vi "Periodic Tasks.vi"(8 "error in":errorcluster) -> ()   [LabVIEW 2020]
doc: "This VI runs in parallel to other tasks. It can contain as many user-defined periodic loops as you need. These can carry out PID or other sorts of timed response."
uses:
  <vilib>/Rock Robotics/WPI/Utilities/WPI_GetSetVariantRefNum.vi
panel:
  out "Temperature Chart":u8(graph)
  out "Output Chart":dbl(graph)
  out "Current Chart":dbl(graph)
  out "Voltage Chart":dbl(graph)
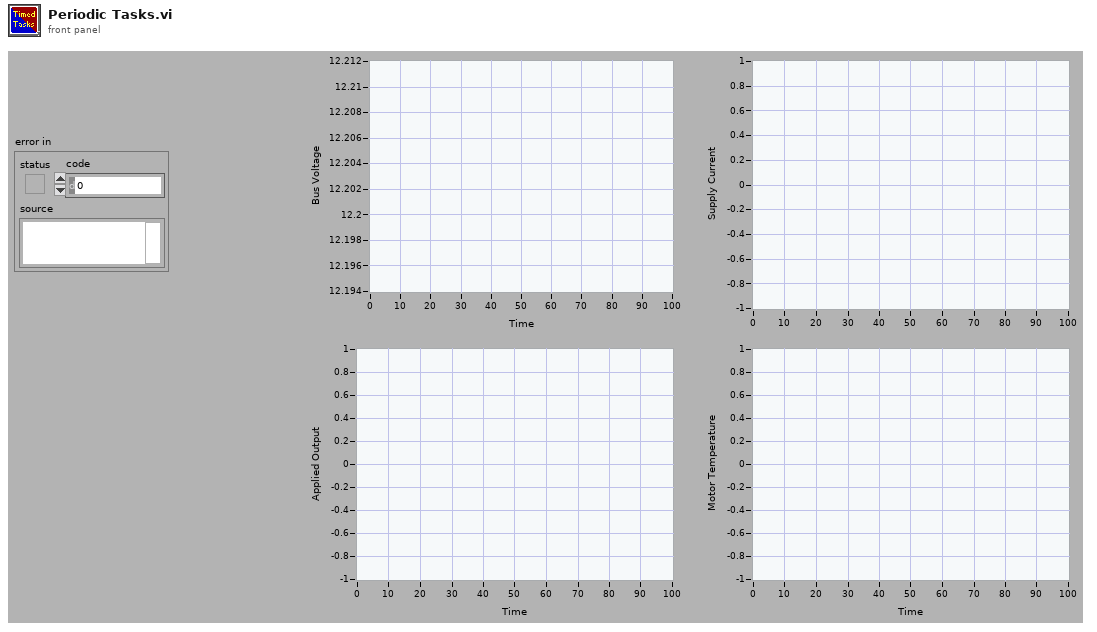
[diagram p1: front panel]
types:
  T1 = typedef "WPI_JoystickDevRef.ctl" = cluster{"Device":T2}
  T2 = typedef "WPI_JoystickDeviceEnum.ctl" = enum16{"USB 0", "USB 1", "USB 2", "USB 3", "USB 4", "USB 5"}
  T3 = typedef "WPI_MotorControlDeviceRef.ctl" = cluster{"DeviceStatus":errorcluster, "Type":T4, "PWM":cluster{"PWM Channel":T5, "DeadBand":T6}, "CAN":cluster{"Device Number":u8, "SetOutput VI Ref":variant, "GetOutput VI Ref":variant, "Enable VI Ref":variant, "Disable VI Ref":variant, "Data":variant}, "Invert":bool, "DIO PWM":cluster{"PWM \"Enable\" Channel":T5, "DIOChannel":T7, "PWM Rate":dbl}}
  T4 = typedef "WPI_MotorControlType.ctl" = enum16{"PWM", "CAN", "DIO PWM"}
  T5 = typedef "FPGA_DIOPWMChannel.ctl" = enum8{"PWM 0", "PWM 1", "PWM 2", "PWM 3", "PWM 4", "PWM 5", "PWM 6", "PWM 7", "PWM 8", "PWM 9", "PWM MXP 0", "PWM MXP 1", "PWM MXP 2", "PWM MXP 3", "PWM MXP 4", "PWM MXP 5", "PWM MXP 6", "PWM MXP 7", "PWM MXP 8", "PWM MXP 9", "Invalid"}
  T6 = typedef "WPI_PWMDeadband.ctl" = cluster{"Name":string, "maxPositivePwm":i32, "minPositivePwm":i32, "centerPwm":i32, "maxNegativePwm":i32, "minNegativePwm":i32, "angularRange":u16}
  T7 = typedef "FPGA_DIOChannel.ctl" = enum8{"DIO 0", "DIO 1", "DIO 2", "DIO 3", "DIO 4", "DIO 5", "DIO 6", "DIO 7", "DIO 8", "DIO 9", "DIO MXP 0", "DIO MXP 1", "DIO MXP 2", "DIO MXP 3", "DIO MXP 4", "DIO MXP 5", "DIO MXP 6", "DIO MXP 7", "DIO MXP 8", "DIO MXP 9", "DIO MXP 10", "DIO MXP 11", "DIO MXP 12", "DIO MXP 13", "DIO MXP 14", "DIO MXP 15", "SPI Port CS1", "SPI Port CS2", "SPI Port CS3", "SPI Port MISO", "SPI Port MOSI", "Invalid"}
  T8 = cluster{"JoystickDevRef":T1, "MotorControlDevRef":T3}
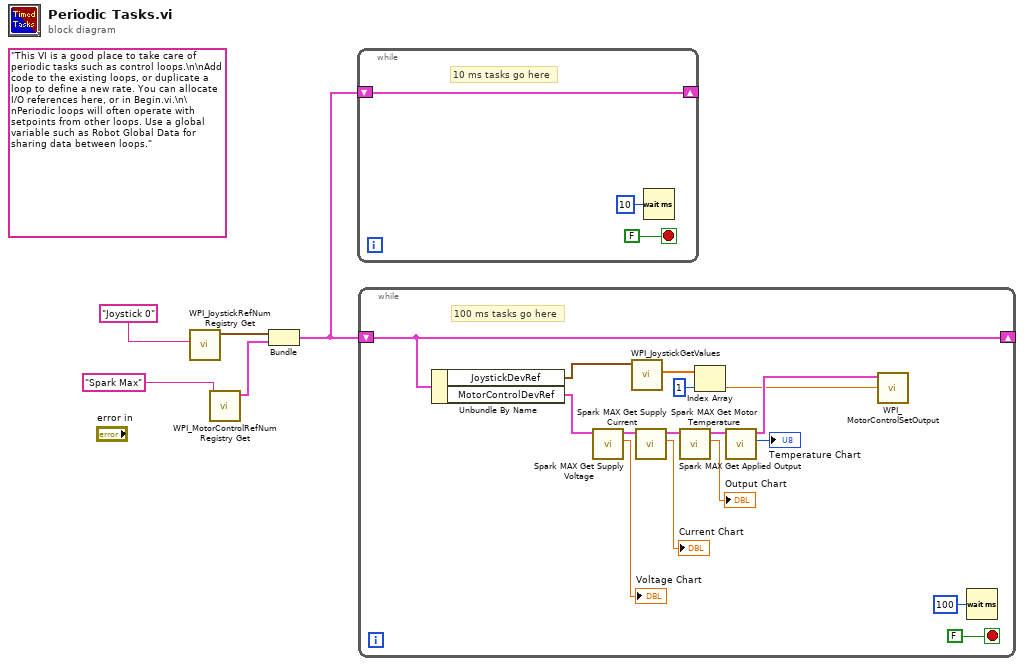
[diagram p0: block diagram]
diagram:
  (unwired) "This VI is a good place to take care of periodic tasks such as control loops.\n\nAdd code to the existing loops, or duplicate a loop to define a new rate. You can allocate I/O references here, or in Begin.vi.\n\nPeriodic loops will often operate with setpoints from other loops. Use a global variable such as Robot Global Data for sharing data between loops."
  n1 = call <vilib>:"WPI_JoystickRefNum Registry Get.vi"("refnum name"="Joystick 0") -> ("JoystickDevRef"=w4:T1)  [unwired: 1 in, 9 out]
  n2 = call <vilib>:"WPI_MotorControlRefNum Registry Get.vi"("refnum name"="Spark Max") -> ("MotorControlDevRef"=w1:T3)  [unwired: 9 in, 1 out]
  n3 = Bundle("JoystickDevRef"=w4, "MotorControlDevRef"=w1) -> (w3:T8)  [unwired: 1 out]
  n4 = while {
    shift-right: [w6] -> _
    shift-left: w3 -> [w6]
    stop <- FALSE stop-if-true
    # "10 ms tasks go here"
    n5 = Wait (ms)(milliseconds to wait=u32 10) -> ()  [unwired: 1 out]
  }
  n6 = while {
    shift-right: [w22] -> _
    shift-left: w3 -> [w22]
    stop <- FALSE stop-if-true
    # "100 ms tasks go here"
    n7 = Unbundle By Name(w22) -> ("JoystickDevRef"=w13:T1, "MotorControlDevRef"=w21:T3)
    n8 = call <vilib>:"Spark MAX Get Supply Voltage.vi"("MotorControlDevRef in"=w21) -> ("Voltage"=→"Voltage Chart":dbl, "MotorControlDevRef out"=w20:T3)  [unwired: 7 in, 2 out]
    n9 = call <vilib>:"WPI_JoystickGetValues.vi"("JoystickDevRef"=w13) -> ("Axes"=w12:dbl[])  [unwired: 6 in, 4 out]
    n10 = call <vilib>:"Spark MAX Get Supply Current.vi"("MotorControlDevRef in"=w20) -> ("Current"=→"Current Chart":dbl, "MotorControlDevRef out"=w19:T3)  [unwired: 7 in, 2 out]
    n11 = call <vilib>:"Spark MAX Get Applied Output.vi"("MotorControlDevRef in"=w19) -> ("Applied Output"=→"Output Chart":dbl, "MotorControlDevRef out"=w15:T3)  [unwired: 7 in, 2 out]
    n12 = Index Array(array=w12, index=1) -> (element=w9:dbl)
    n13 = call <vilib>:"Spark MAX Get Motor Temperature.vi"("MotorControlDevRef in"=w15) -> ("Motor Temperature"=→"Temperature Chart":u8, "MotorControlDevRef out"=w10:T3)  [unwired: 7 in, 2 out]
    n14 = call <vilib>:"WPI_MotorControlSetOutput.vi"("Output"=w9, "MotorControlDevRef"=w10) -> ()  [unwired: 7 in, 3 out]
    n15 = Wait (ms)(milliseconds to wait=u32 100) -> ()  [unwired: 1 out]
  }
